vi "Command Settings.vi"() -> (5 "Command Settings":T1[](array[typedef])=[{"Enum"=enum."Update Data", "U8"=0, " Payload"=TRUE}, {"Enum"=enum."Update Data", "U8"=0, " Payload"=FALSE}, {"Enum"=enum."Update Data", "U8"=0, " Payload"=TRUE}, {"Enum"=enum."Update Data", "U8"=0, " Payload"=TRUE}, {"Enum"=enum."Update Data", "U8"=0, " Payload"=TRUE}, {"Enum"=enum."Update Data", "U8"=0, " Payload"=FALSE}, {"Enum"=enum."Update Data", "U8"=0, " Payload"=TRUE}, {"Enum"=enum."Update Data", "U8"=0, " Payload"=FALSE}, {"Enum"=enum."Update Data", "U8"=0, " Payload"=FALSE}, {"Enum"=enum."Update Data", "U8"=0, " Payload"=FALSE}])   [LabVIEW 2021, in "CIFCustomOOB_Tx.lvclass"]
uses:
  CIFCustomOOB_Tx.lvclass
  Typedef/Command Setting Control.ctl
  Typedef/OOB Commands.ctl
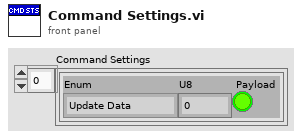
[diagram p1: front panel]
types:
  T1 = typedef "CIFCustomOOB_Tx.lvclass/Command Setting Control.ctl" = cluster{"Enum":T2, "U8":u8, " Payload":bool}
  T2 = typedef "CIFCustomOOB_Tx.lvclass/OOB Commands.ctl" = enum8{"Update Data"}
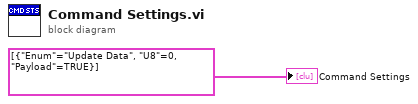
[diagram p0: block diagram]
diagram:
  "Command Settings" <- cluster{"Enum":T2, "U8":u8, "Payload":bool}[] [{"Enum"=enum."Update Data", "U8"=0, "Payload"=TRUE}]
